vi "Write Single Holding Register.vi"(8 "error in (no error)":errorcluster, 9 "value":u16, 10 "address":u16, 11 "MODBUS in":refnum<class "Modbus.lvclass">) -> (0 "error out":errorcluster, 3 "MODBUS Out":refnum<class "Modbus.lvclass">)   [LabVIEW 2020, in "Library Instrument & Equipement.lvlib" / "Library Relay_Board.lvlib" / "Modbus.lvclass"]
doc: "Writes single holding register <B>value</B> at specified <B>address</B> (Modbus function code: <B>6</B>)."
uses:
  Modbus.lvclass
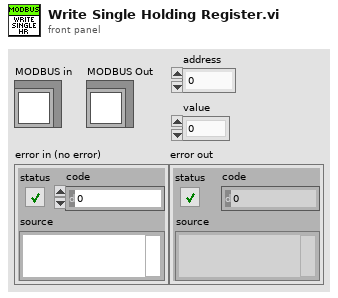
[diagram p1: front panel]
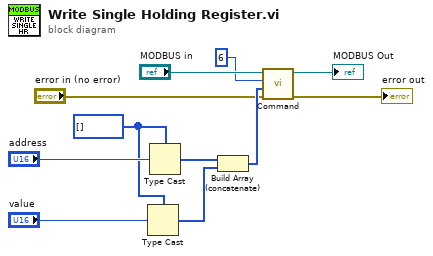
[diagram p0: block diagram]
diagram:
  w4 = u8[] []
  n1 = Type Cast(type=w4, x="value") -> (*(type *) &x=w8:u8[])
  n2 = Type Cast(type=w4, x="address") -> (*(type *) &x=w9:u8[])
  n3 = Build Array (concatenate)(w9, w8) -> (w7:u8[])
  n4 = call-dynamic "Command.vi"("error in (no error)"="error in (no error)", "data in"=w7, "function code"=u8 6 ("function"), "MODBUS in"="MODBUS in") -> ("error out"=→"error out":errorcluster, "MODBUS Out"=→"MODBUS Out":refnum<class "Modbus.lvclass">)  [unwired: 5 in, 1 out]
